vi "libssh2_sftp_shutdown.vi"(8 "error in (no error)":errorcluster, 11 "sftp":T1) -> (0 "error out":errorcluster)   [LabVIEW 2013, in "libssh2.lvlib"]
doc: "Shutdown an SFTP session."
uses:
  libssh2.lvlib
  SFTP Refnum.ctl
  Global Settings.vi
  Read Session Refnum.vi
  <vilib>/Utility/semaphor.llb/Acquire Semaphore.vi
  <vilib>/Utility/semaphor.llb/Release Semaphore.vi
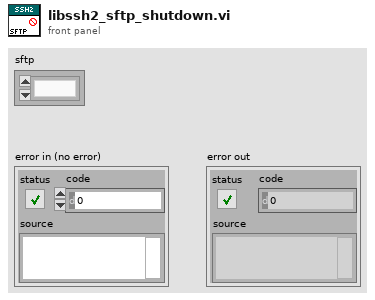
[diagram p1: front panel]
types:
  T1 = typedef "libssh2.lvlib/SFTP Refnum.ctl" = refnum<k1>
  T2 = typedef "libssh2.lvlib/Session Refnum.ctl" = refnum<k1>
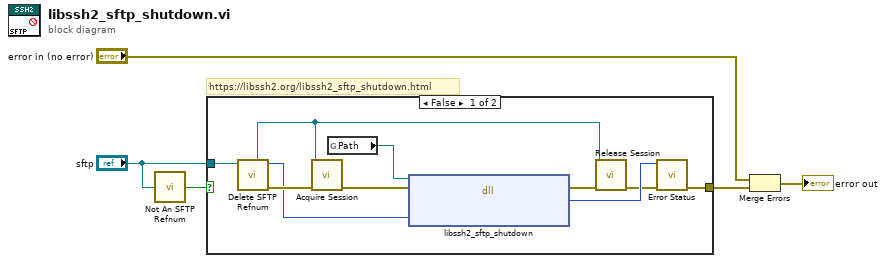
[diagram p0: block diagram]
diagram:
  # "https://libssh2.org/libssh2_sftp_shutdown.html"
  n1 = call "Not An SFTP Refnum.vi"("sftp"="sftp") -> ("Not a SFTP Refnum?"=w5:bool)
  n2 = case shown="False" w5 {
    tunnel: "sftp" -> [w14 _]
    tunnel: [w10 _] -> w4
    frame False {
      n3 = call "Delete SFTP Refnum.vi"("sftp"=w14) -> ("error out"=w13:errorcluster, "LIBSSH2_SFTP*"=w12:u64, "session"=w6:T2)  [unwired: 8 in]
      n4 = call "Acquire Session.vi"("error in (no error)"=w13, "session"=w6) -> ("error out"=w8:errorcluster)  [unwired: 7 in, 2 out]
      n5 = global read "Global Settings.vi" "Path"() -> (w15:path)
      n6 = dll-call lib="?" fn="libssh2_sftp_shutdown"(path in=w15, error in=w8, "sftp"=w12) -> (error out=w11:errorcluster, "return value"=w9:i32)  [unwired: 2 in, 1 out]
      n7 = call "Release Session.vi"("error in (no error)"=w11, "session"=w6) -> ("error out"=w7:errorcluster)  [unwired: 9 in]
      n8 = call "Error Status.vi"("error in (no error)"=w7, "return value"=w9) -> ("error out"=w10:errorcluster)  [unwired: 8 in, 1 out]
    }
    frame True {
    }
  }
  n9 = Merge Errors("error in (no error)", w4) -> (→"error out":errorcluster)
